vi "pubsub.vi"() -> ()   [LabVIEW 2015]
uses:
  publisher/publisher.lvclass
  subscriber.lvclass
  client/connection client.lvclass/connection client.ctl
  communicator/communicator.lvclass/communicator.ctl
  communicator queue/identifying queue.lvclass/identifying queue.ctl
  message/communicator message.lvclass/communicator message.ctl
  client/prepare client.vi
  server/prepare server.vi
  message/set sender.vi
  TCP/TCP server.lvclass
  TCP client/TCP client.lvclass
  communicator queue/identifying queue.lvclass
  message/communicator message.lvclass
  communicator/communicator.lvclass
  manager/queue manager.lvclass
  communicator manager/communicator manager.lvlib
panel:
  out "pubID 2":string
  out "pubData 2":variant
  out "subData 2":variant
  out "subID 2":string
  in  "publish":bool
  in  "pubstringdata":string
  in  "pubStringID":string
  in  "destroysub":bool
  in  "createsub":bool
  in  "subscription":string
  in  "stop":bool
  out "subData":variant
  out "subID":string
  out "pubID":string
  out "pubData":variant
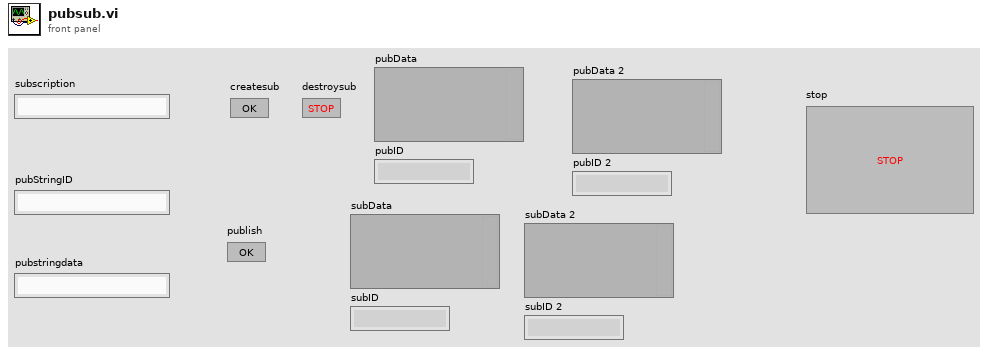
[diagram p1: front panel]
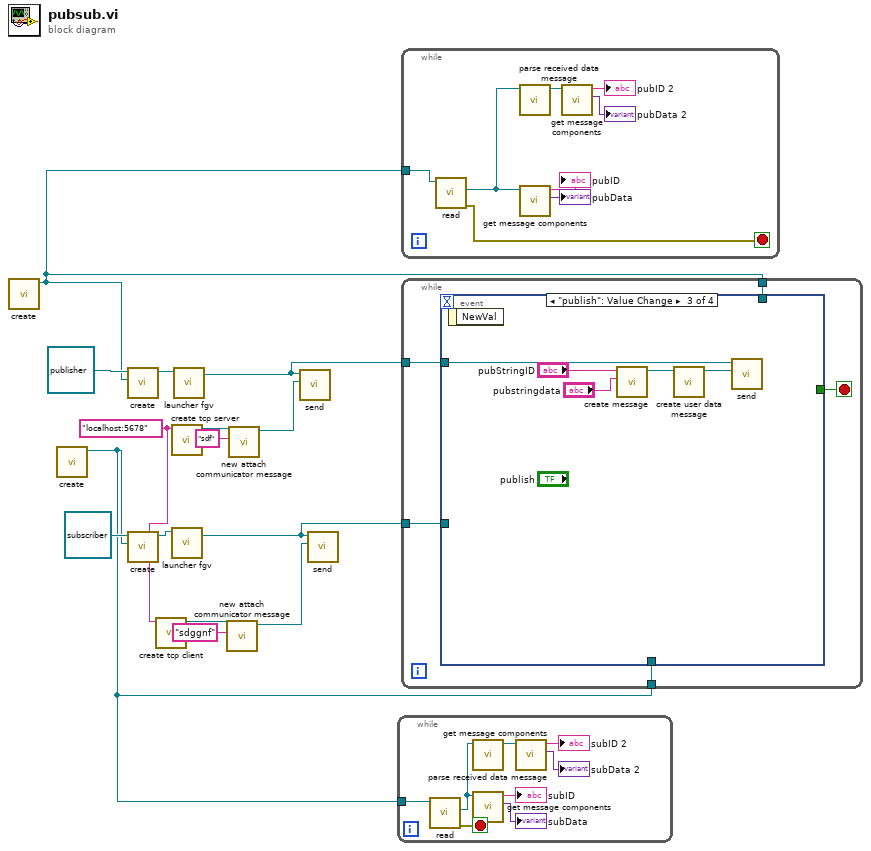
[diagram p0: block diagram]
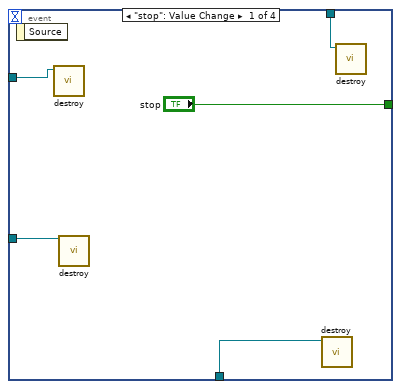
[diagram p2: hidden frame]
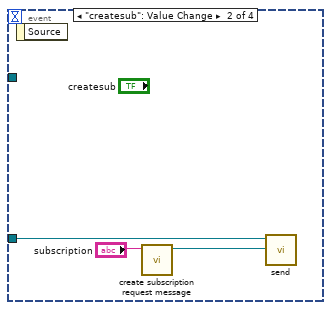
[diagram p3: hidden frame]
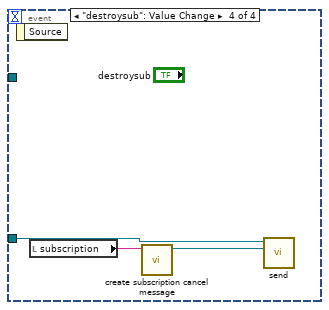
[diagram p4: hidden frame]
diagram:
  w9 = "localhost:5678" ("conn string")
  n1 = call "create.vi"() -> ("message connection out"=w4:refnum<class "identifying queue.lvclass">)  [unwired: 10 in, 1 out]
  n2 = call "create.vi"() -> ("message connection out"=w3:refnum<class "identifying queue.lvclass">)  [unwired: 10 in, 1 out]
  n3 = call "create.vi"("parent"=w4, "uninitialized communicator"=refnum<class "publisher.lvclass"> refnum ("publisher")) -> ("communicator out"=w6:refnum<class "publisher.lvclass">)  [unwired: 8 in, 1 out]
  n4 = call "create.vi"("parent"=w3, "uninitialized communicator"=refnum<class "subscriber.lvclass"> refnum ("subscriber")) -> ("communicator out"=w5:refnum<class "subscriber.lvclass">)  [unwired: 8 in, 1 out]
  n5 = call "create tcp client.vi"("conn string"=w9) -> ("TCP client out"=w13:refnum<class "TCP client.lvclass">)  [unwired: 9 in, 1 out]
  n6 = call "create tcp server.vi"("conn string"=w9) -> ("TCP server out"=w12:refnum<class "TCP server.lvclass">)  [unwired: 9 in, 1 out]
  n7 = call "launcher fgv.vi"("communicator in"=w5) -> ("initialized communicator"=w7:refnum<class "communicator.lvclass">)  [unwired: 9 in, 1 out]
  n8 = call "launcher fgv.vi"("communicator in"=w6) -> ("initialized communicator"=w8:refnum<class "communicator.lvclass">)  [unwired: 9 in, 1 out]
  n9 = call "new attach communicator message.vi"("ID"="sdggnf", "comm"=w13) -> ("message"=w10:refnum<class "communicator message.lvclass">)  [unwired: 9 in]
  n10 = call "new attach communicator message.vi"("ID"="sdf", "comm"=w12) -> ("message"=w11:refnum<class "communicator message.lvclass">)  [unwired: 9 in]
  n11 = call "send.vi"("element"=w11, "communicator in"=w8) -> ()  [unwired: 9 in, 1 out]
  n12 = call "send.vi"("element"=w10, "communicator in"=w7) -> ()  [unwired: 9 in, 1 out]
  n13 = while {
    tunnel: w3 -> [w23]
    stop <- w22 stop-if-true
    n14 = call "read.vi"("identifying queue in"=w23) -> ("error out"=w22:errorcluster, "message"=w18:refnum<class "communicator message.lvclass">)  [unwired: 8 in, 1 out]
    n15 = call "parse received data message.vi"("message"=w18) -> ("data"=w19:refnum<class "communicator message.lvclass">)  [unwired: 9 in, 1 out]
    n16 = call "get message components.vi"("message"=w18) -> ("data"=→"subData":variant, "ID"=→"subID":string)  [unwired: 9 in]
    n17 = call "get message components.vi"("message"=w19) -> ("data"=→"subData 2":variant, "ID"=→"subID 2":string)  [unwired: 9 in]
  }
  n18 = while {
    tunnel: w4 -> [w31]
    stop <- w30 stop-if-true
    n19 = call "read.vi"("identifying queue in"=w31) -> ("error out"=w30:errorcluster, "message"=w24:refnum<class "communicator message.lvclass">)  [unwired: 8 in, 1 out]
    n20 = call "parse received data message.vi"("message"=w24) -> ("data"=w27:refnum<class "communicator message.lvclass">)  [unwired: 9 in, 1 out]
    n21 = call "get message components.vi"("message"=w24) -> ("data"=→"pubData":variant, "ID"=→"pubID":string)  [unwired: 9 in]
    n22 = call "get message components.vi"("message"=w27) -> ("data"=→"pubData 2":variant, "ID"=→"pubID 2":string)  [unwired: 9 in]
  }
  n23 = while {
    tunnel: w8 -> [w34]
    tunnel: w7 -> [w35]
    tunnel: w4 -> [w33]
    tunnel: w3 -> [w32]
    stop <- w36 stop-if-true
    n24 = event shown="[2] \"publish\": Value Change" {
      selector: _ -> [_ _ _ _]
      dyn-events: _ -> [_ _ _ _]
      timeout: _ -> [_ _ _ _]
      tunnel: ["stop" _ _ _] -> w36
      tunnel: w35 -> [w39 w44 _ w52]
      tunnel: w34 -> [w40 _ w49 _]
      tunnel: w33 -> [w38 _ _ _]
      tunnel: w32 -> [w37 _ _ _]
      event "stop": Value Change {
        n25 = event-data() -> ()  [unwired: 1 in, 1 out]
        n26 = call-dynamic "destroy.vi"("communicator in"=w40) -> ()  [unwired: 10 in, 1 out]
        n27 = call-dynamic "destroy.vi"("communicator in"=w39) -> ()  [unwired: 10 in, 1 out]
        n28 = call "destroy.vi"("message connection in"=w37) -> ()  [unwired: 10 in, 1 out]
        n29 = call "destroy.vi"("message connection in"=w38) -> ()  [unwired: 10 in, 1 out]
      }
      event "createsub": Value Change {
        n30 = event-data() -> ()  [unwired: 1 in, 1 out]
        n31 = call "create subscription request message.vi"("pattern"="subscription") -> ("message"=w43:refnum<class "communicator message.lvclass">)  [unwired: 10 in]
        n32 = call "send.vi"("element"=w43, "communicator in"=w44) -> ()  [unwired: 9 in, 1 out]
      }
      event "publish": Value Change {
        n33 = event-data() -> ()  [unwired: 1 in, 1 out]
        n34 = call "create message.vi"("data"="pubstringdata", "ID"="pubStringID") -> ("message"=w48:refnum<class "communicator message.lvclass">)  [unwired: 9 in]
        n35 = call "create user data message.vi"("data"=w48) -> ("message"=w45:refnum<class "communicator message.lvclass">)  [unwired: 10 in]
        n36 = call "send.vi"("element"=w45, "communicator in"=w49) -> ()  [unwired: 9 in, 1 out]
      }
      event "destroysub": Value Change {
        n37 = event-data() -> ()  [unwired: 1 in, 1 out]
        n38 = local read "subscription"() -> (w50:string)
        n39 = call "create subscription cancel message.vi"("pattern"=w50) -> ("message"=w51:refnum<class "communicator message.lvclass">)  [unwired: 10 in]
        n40 = call "send.vi"("element"=w51, "communicator in"=w52) -> ()  [unwired: 9 in, 1 out]
      }
    }
  }
